vi "dimensions.vi"() -> ()   [LabVIEW 2015, in "Build JSON Array.xnode"]
uses:
  Build JSON Array.xnode
panel:
  in  "footer.h":i16=8
  in  "element.h":i16=8
  in  "resize.v":i32=8
  in  "min.h":i32=16
  in  "min.w":i32=32
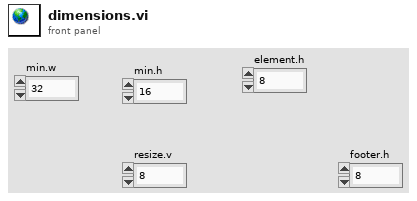
[diagram p1: front panel]
diagram:
